vi "Errorbar2009.vi"   [LabVIEW 2013]
uses:
  <vilib>/Heliosphere Research LLC/Advanced Plotting Toolkit/Advanced Plotting Toolkit.lvlib
types:
  T1 = typedef "Advanced Plotting Toolkit.lvlib/PlotID.ctl" = i32
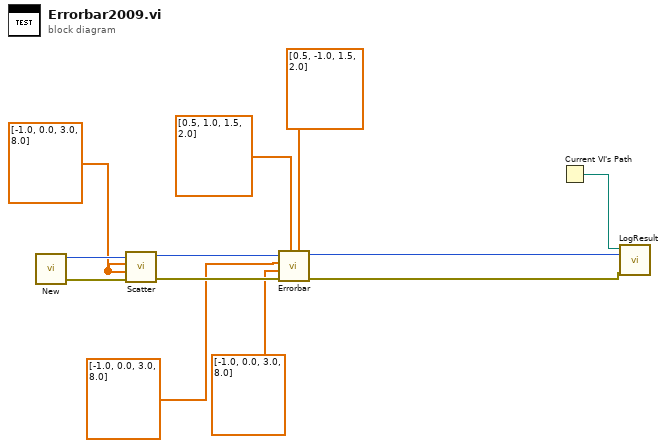
[diagram p0: block diagram]
diagram:
  w5 = dbl[] [-1.0, 0.0, 3.0, 8.0] ("X Data")
  n1 = call <vilib>:"New.vi"() -> ("error out"=w6:errorcluster, "Plot ID"=w9:T1)  [unwired: 10 in]
  n2 = call <vilib>:"Scatter.vi"("error in (no error)"=w6, "Y Data"=w5, "X Data"=w5, "Plot ID"=w9) -> ("error out"=w7:errorcluster, "Plot ID Out"=w8:T1)  [unwired: 6 in]
  n3 = call <vilib>:"Errorbar.vi"("Y Errors"=dbl[] [0.5, -1.0, 1.5, 2.0] ("X Errors"), "X Errors"=dbl[] [0.5, 1.0, 1.5, 2.0], "error in (no error)"=w7, "Y Data"=dbl[] [-1.0, 0.0, 3.0, 8.0] ("X Data"), "X Data"=dbl[] [-1.0, 0.0, 3.0, 8.0], "Plot ID"=w8) -> ("error out"=w10:errorcluster, "Plot ID out"=w11:T1)  [unwired: 4 in]
  n4 = Current VI's Path() -> (path=w12:path)
  n5 = call "LogResult.vi"("Test Result"=w10, "Test Artifact"=w11, "VI Path"=w12) -> ()  [unwired: 9 in]
